vi "svx_Colormap ReplaceState.vi"(9 "Events":T2[](array[typedef])=[enum."[Data] Update"], 10 "RefState":T1={"RefQueue"=refnum, "Properties/Undo"=refnum, "Bound"={"Width"=0, "Height"=0}, "Plot Area:Colors"={"FG Color"=11776947, "BG Color"=0}, "scale legend visible?"=FALSE, "graph palette visible?"=FALSE, "cursor palette visible?"=FALSE, "Ignore Array"=TRUE, "Smooth Update"=FALSE, "Z Scale"={"Z Scale.Scale Fit"=2, "Z Scale.Name Label.Text"="Amplitude", "Z Scale.Interpolate Color"=TRUE, "Visible"=TRUE, "Label Visible"=TRUE, "format string"="%#.2g", "Z Scale.Range"={"Minimum"=0.0, "Maximum"=500.0}}, "X Scale"={"X Scale.Scale Fit"=2, "X Scale.Offset and Multiplier"={"Offset"=0.0, "Multiplier"=1.0}, "X Scale.Name Label.Text"="Time", "X Scale.Range"={"Minimum"=0.0, "Maximum"=10.0}, "Visible"=TRUE, "Label Visible"=TRUE, "format string"="%#.2g"}, "Y Scale"={"Y Scale.Scale Fit"=2, "Y Scale.Offset and Multiplier"={"Offset"=0.0, "Multiplier"=1.0}, "Y Scale.Name Label.Text"="Frequency", "Y Scale.Range"={"Minimum"=0.0, "Maximum"=500.0}, "Visible"=TRUE, "Label Visible"=TRUE, "format string"="%#.2g"}, "Annotation List"=[], "Cursor List"=[], "Display Frequency Lines"=TRUE, "Display Order Lines"=TRUE, "Display Order text"=TRUE, "Display Frequency text"=TRUE, "Order Lineproperty"={"Line"={"Width"=1, "Style"=enum."Dash"}, "color"=0}, "Order Textproperty"={"Test size"=11, "color"=16777222, "background"=16777216}, "Orders"=[], "Frequency"=[], "Frequency Lineproperty"={"Line"={"Width"=1, "Style"=enum."Dash"}, "color"=0}, "Frequency Textproperty"={"Test size"=11, "color"=16777222, "background"=16777216}, "Display Order from Cursor"=FALSE, "Display Freq from Cursor"=FALSE, "Active Cursor"=0, "Selected Cursors"=[], "Cursor Move"=refnum, "Scale Range Change"=refnum}, 11 "NewState":T1={"RefQueue"=refnum, "Properties/Undo"=refnum, "Bound"={"Width"=0, "Height"=0}, "Plot Area:Colors"={"FG Color"=11776947, "BG Color"=0}, "scale legend visible?"=FALSE, "graph palette visible?"=FALSE, "cursor palette visible?"=FALSE, "Ignore Array"=TRUE, "Smooth Update"=FALSE, "Z Scale"={"Z Scale.Scale Fit"=2, "Z Scale.Name Label.Text"="Amplitude", "Z Scale.Interpolate Color"=TRUE, "Visible"=TRUE, "Label Visible"=TRUE, "format string"="%#.2g", "Z Scale.Range"={"Minimum"=0.0, "Maximum"=500.0}}, "X Scale"={"X Scale.Scale Fit"=2, "X Scale.Offset and Multiplier"={"Offset"=0.0, "Multiplier"=1.0}, "X Scale.Name Label.Text"="Time", "X Scale.Range"={"Minimum"=0.0, "Maximum"=10.0}, "Visible"=TRUE, "Label Visible"=TRUE, "format string"="%#.2g"}, "Y Scale"={"Y Scale.Scale Fit"=2, "Y Scale.Offset and Multiplier"={"Offset"=0.0, "Multiplier"=1.0}, "Y Scale.Name Label.Text"="Frequency", "Y Scale.Range"={"Minimum"=0.0, "Maximum"=500.0}, "Visible"=TRUE, "Label Visible"=TRUE, "format string"="%#.2g"}, "Annotation List"=[], "Cursor List"=[], "Display Frequency Lines"=TRUE, "Display Order Lines"=TRUE, "Display Order text"=TRUE, "Display Frequency text"=TRUE, "Order Lineproperty"={"Line"={"Width"=1, "Style"=enum."Dash"}, "color"=0}, "Order Textproperty"={"Test size"=11, "color"=16777222, "background"=16777216}, "Orders"=[], "Frequency"=[], "Frequency Lineproperty"={"Line"={"Width"=1, "Style"=enum."Dash"}, "color"=0}, "Frequency Textproperty"={"Test size"=11, "color"=16777222, "background"=16777216}, "Display Order from Cursor"=FALSE, "Display Freq from Cursor"=FALSE, "Active Cursor"=0, "Selected Cursors"=[], "Cursor Move"=refnum, "Scale Range Change"=refnum}) -> (3 "State out":T1={"RefQueue"=refnum, "Properties/Undo"=refnum, "Bound"={"Width"=0, "Height"=0}, "Plot Area:Colors"={"FG Color"=11776947, "BG Color"=0}, "scale legend visible?"=FALSE, "graph palette visible?"=FALSE, "cursor palette visible?"=FALSE, "Ignore Array"=TRUE, "Smooth Update"=FALSE, "Z Scale"={"Z Scale.Scale Fit"=2, "Z Scale.Name Label.Text"="Amplitude", "Z Scale.Interpolate Color"=TRUE, "Visible"=TRUE, "Label Visible"=TRUE, "format string"="%#.2g", "Z Scale.Range"={"Minimum"=0.0, "Maximum"=500.0}}, "X Scale"={"X Scale.Scale Fit"=2, "X Scale.Offset and Multiplier"={"Offset"=0.0, "Multiplier"=1.0}, "X Scale.Name Label.Text"="Time", "X Scale.Range"={"Minimum"=0.0, "Maximum"=10.0}, "Visible"=TRUE, "Label Visible"=TRUE, "format string"="%#.2g"}, "Y Scale"={"Y Scale.Scale Fit"=2, "Y Scale.Offset and Multiplier"={"Offset"=0.0, "Multiplier"=1.0}, "Y Scale.Name Label.Text"="Frequency", "Y Scale.Range"={"Minimum"=0.0, "Maximum"=500.0}, "Visible"=TRUE, "Label Visible"=TRUE, "format string"="%#.2g"}, "Annotation List"=[], "Cursor List"=[], "Display Frequency Lines"=TRUE, "Display Order Lines"=TRUE, "Display Order text"=TRUE, "Display Frequency text"=TRUE, "Order Lineproperty"={"Line"={"Width"=1, "Style"=enum."Dash"}, "color"=0}, "Order Textproperty"={"Test size"=11, "color"=16777222, "background"=16777216}, "Orders"=[], "Frequency"=[], "Frequency Lineproperty"={"Line"={"Width"=1, "Style"=enum."Dash"}, "color"=0}, "Frequency Textproperty"={"Test size"=11, "color"=16777222, "background"=16777216}, "Display Order from Cursor"=FALSE, "Display Freq from Cursor"=FALSE, "Active Cursor"=0, "Selected Cursors"=[], "Cursor Move"=refnum, "Scale Range Change"=refnum})   [LabVIEW 2017, in "SVX Colormap.xctl"]
uses:
  <vilib>/addons/_XControls/Colormap/SVX Colormap.xctl
  <vilib>/addons/_XControls/Colormap/TypeDef/svx_Colormap_Event.ctl
  <vilib>/addons/_XControls/Colormap/subVIs/svx_Colormap State.ctl
  <vilib>/addons/_XControls/Colormap/TypeDef/svx_Colormap_InnerState.ctl
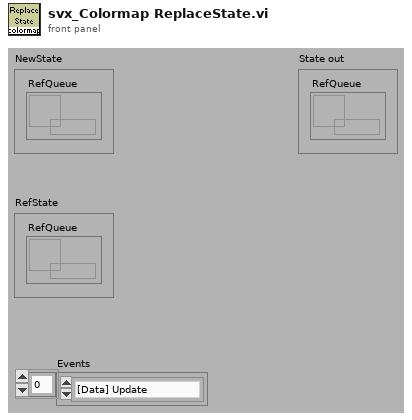
[diagram p1: front panel]
types:
  T1 = typedef "SVX Colormap.xctl/svx_Colormap State.ctl" = cluster{"RefQueue":refnum<queue>, "Properties/Undo":refnum<queue>, "Bound":cluster{"Width":u32, "Height":u32}, "Plot Area:Colors":cluster{"FG Color":u32, "BG Color":u32}, "scale legend visible?":bool, "graph palette visible?":bool, "cursor palette visible?":bool, "Ignore Array":bool, "Smooth Update":bool, "Z Scale":cluster{"Z Scale.Scale Fit":u8, "Z Scale.Name Label.Text":string, "Z Scale.Interpolate Color":bool, "Visible":bool, "Label Visible":bool, "format string":string, "Z Scale.Range":cluster{"Minimum":dbl, "Maximum":dbl}}, "X Scale":cluster{"X Scale.Scale Fit":u8, "X Scale.Offset and Multiplier":cluster{"Offset":dbl, "Multiplier":dbl}, "X Scale.Name Label.Text":string, "X Scale.Range":cluster{"Minimum":dbl, "Maximum":dbl}, "Visible":bool, "Label Visible":bool, "format string":string}, "Y Scale":cluster{"Y Scale.Scale Fit":u8, "Y Scale.Offset and Multiplier":cluster{"Offset":dbl, "Multiplier":dbl}, "Y Scale.Name Label.Text":string, "Y Scale.Range":cluster{"Minimum":dbl, "Maximum":dbl}, "Visible":bool, "Label Visible":bool, "format string":string}, "Annotation List":cluster{"Name":string, "Color":u32, "Style":u8, "Point Style":u8, "Name Visible":bool, "Allow Drag":bool, "Annotation Mode":u32, "Plot":i32, "Index":i32, "Position":cluster{"X":dbl, "Y":dbl}, "X Scale":u32, "Y Scale":u32, "Show Arrow":bool, "Lock Name":bool, "Plot Area":i32, "Label Offset":cluster{"X":dbl, "Y":dbl}}[], "Cursor List":cluster{"Name":string, "Color":u32, "Style":u8, "Point Style":u8, "Name Visible":bool, "Allow Drag":bool, "Cursor Mode":u32, "Plot":i32, "Index":i32, "Position":cluster{"X":dbl, "Y":dbl}, "X Scale":u32, "Y Scale":u32, "Watch Plots":i32[], "Watch All Plots":bool, "Plot Area":i32, "Label Offset":cluster{"X":dbl, "Y":dbl}}[], "Display Frequency Lines":bool, "Display Order Lines":bool, "Display Order text":bool, "Display Frequency text":bool, "Order Lineproperty":cluster{"Line":cluster{"Width":u16, "Style":enum32{"Solid", "Dash", "Dot", "DashDot", "DashDotDot"}}, "color":u32}, "Order Textproperty":cluster{"Test size":i16, "color":u32, "background":u32}, "Orders":dbl[], "Frequency":dbl[], "Frequency Lineproperty":cluster{"Line":cluster{"Width":u16, "Style":enum32{"Solid", "Dash", "Dot", "DashDot", "DashDotDot"}}, "color":u32}, "Frequency Textproperty":cluster{"Test size":i16, "color":u32, "background":u32}, "Display Order from Cursor":bool, "Display Freq from Cursor":bool, "Active Cursor":u32, "Selected Cursors":u32[], "Cursor Move":refnum<user-event>, "Scale Range Change":refnum<user-event>}
  T2 = typedef "SVX Colormap.xctl/svx_Colormap_Event.ctl" = enum16{"None", "[Axis] X Range", "[Axis] Y Range", "[Axis] Z Range", "[Axis] Range", "[Axis] X FString", "[Axis] Y FString", "[Axis] Z FString", "[Axis] X Name", "[Axis] X ScaleVis", "[Axis] X NameVis", "[Axis] Y Name", "[Axis] Y ScaleVis", "[Axis] Y NameVis", "[Axis] Z Name", "[Axis] Z ScaleVis", "[Axis] Z NameVis", "[Image] Line", "[Axis] Z Interp", "[Data] Update", "[Layout] Resize", "[ColorTable] Ignore Array", "[Legend] ScaleVis", "[Legend] GPVis", "[Legend] CPVis", "[Smooth] Update", "[Cursor] Update", "[Plot Area] Colors", "[Size] Minimum", "[Annotation] Update", "[Properties Dialog]", "[Axis] Autoscale X", "[Axis] Autoscale Y", "[Axis] Autoscale Z"}
  T3 = cluster{"Line":cluster{"Width":u16, "Style":enum32{"Solid", "Dash", "Dot", "DashDot", "DashDotDot"}}, "color":u32}
  T4 = cluster{"Test size":i16, "color":u32, "background":u32}
  T5 = cluster{"Name":string, "Color":u32, "Style":u8, "Point Style":u8, "Name Visible":bool, "Allow Drag":bool, "Cursor Mode":u32, "Plot":i32, "Index":i32, "Position":cluster{"X":dbl, "Y":dbl}, "X Scale":u32, "Y Scale":u32, "Watch Plots":i32[], "Watch All Plots":bool, "Plot Area":i32, "Label Offset":cluster{"X":dbl, "Y":dbl}}[]
  T6 = cluster{"Z Scale.Scale Fit":u8, "Z Scale.Name Label.Text":string, "Z Scale.Interpolate Color":bool, "Visible":bool, "Label Visible":bool, "format string":string, "Z Scale.Range":cluster{"Minimum":dbl, "Maximum":dbl}}
  T7 = cluster{"X Scale.Scale Fit":u8, "X Scale.Offset and Multiplier":cluster{"Offset":dbl, "Multiplier":dbl}, "X Scale.Name Label.Text":string, "X Scale.Range":cluster{"Minimum":dbl, "Maximum":dbl}, "Visible":bool, "Label Visible":bool, "format string":string}
  T8 = cluster{"Y Scale.Scale Fit":u8, "Y Scale.Offset and Multiplier":cluster{"Offset":dbl, "Multiplier":dbl}, "Y Scale.Name Label.Text":string, "Y Scale.Range":cluster{"Minimum":dbl, "Maximum":dbl}, "Visible":bool, "Label Visible":bool, "format string":string}
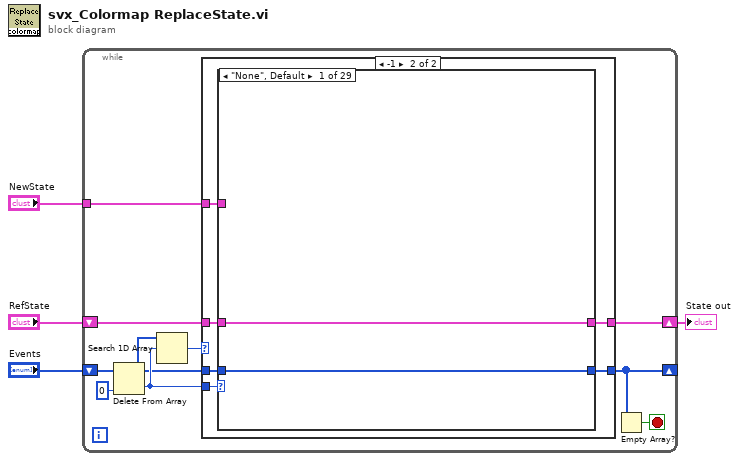
[diagram p0: block diagram]
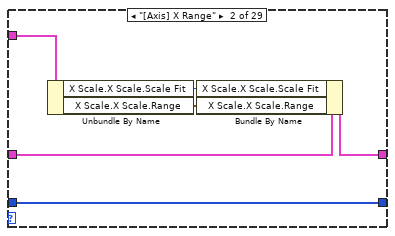
[diagram p3: hidden frame]
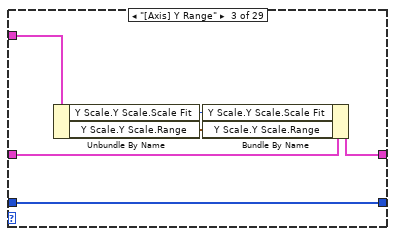
[diagram p4: hidden frame]
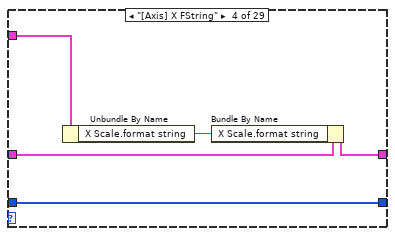
[diagram p5: hidden frame]
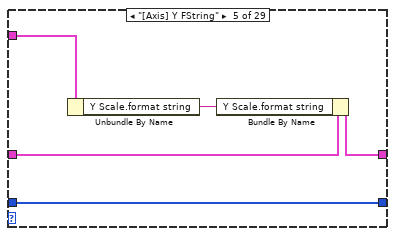
[diagram p6: hidden frame]
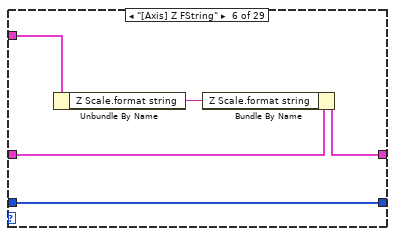
[diagram p7: hidden frame]
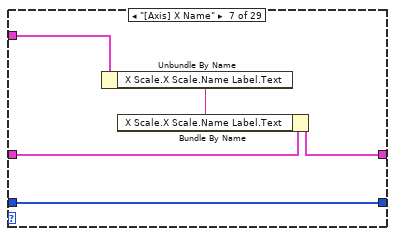
[diagram p8: hidden frame]
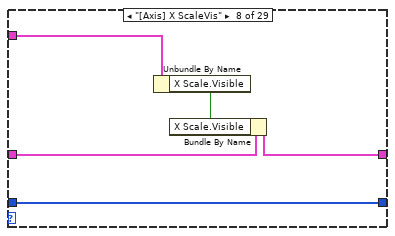
[diagram p9: hidden frame]
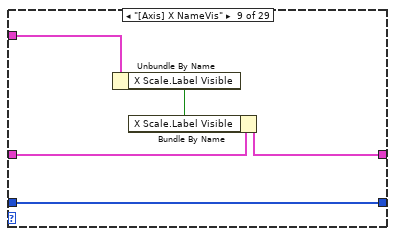
[diagram p10: hidden frame]
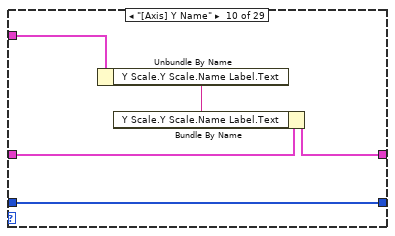
[diagram p11: hidden frame]
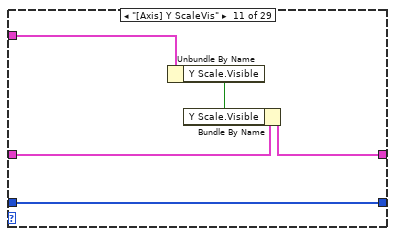
[diagram p12: hidden frame]
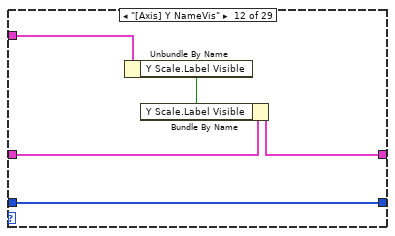
[diagram p13: hidden frame]
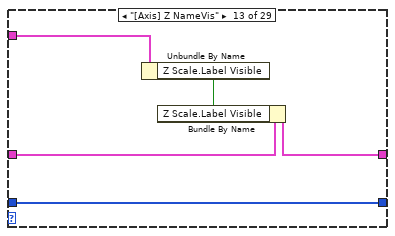
[diagram p14: hidden frame]
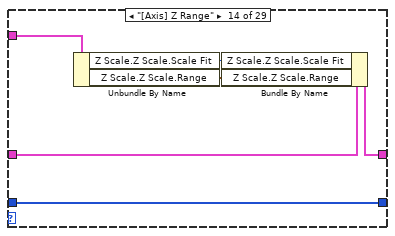
[diagram p15: hidden frame]
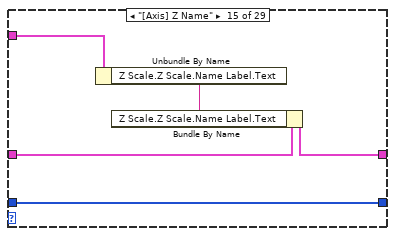
[diagram p16: hidden frame]
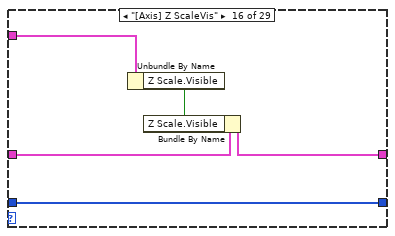
[diagram p17: hidden frame]
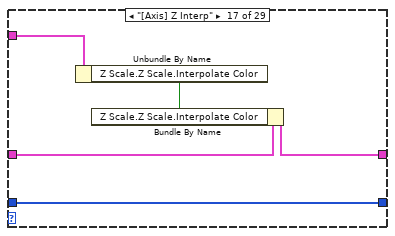
[diagram p18: hidden frame]
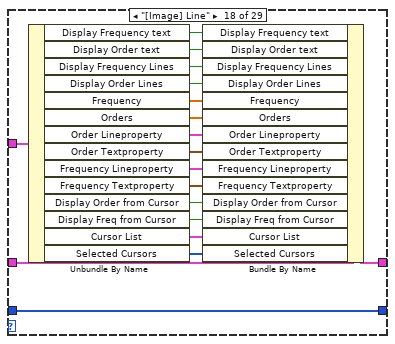
[diagram p19: hidden frame]
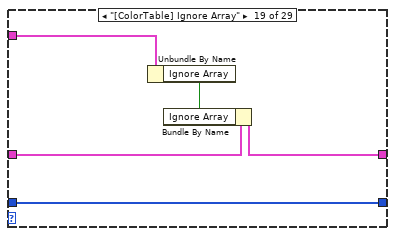
[diagram p20: hidden frame]
diagram:
  n1 = while {
    shift-right: [w9] -> w1
    shift-left: "RefState" -> [w14]
    shift-right: [w11] -> _
    shift-left: "Events" -> [w12]
    tunnel: "NewState" -> [w5]
    stop <- w10 stop-if-true
    n2 = Delete From Array(array=w12, index=0) -> (deleted portion=w8:T2, array with subset deleted=w7:T2[])  [unwired: 1 in]
    n3 = Search 1D Array(1D array=w7, element=w8) -> (index of element=w6:i32)  [unwired: 1 in]
    n4 = case shown="-1" w6 {
      tunnel: w14 -> [w16 w22]
      tunnel: [w15 w21] -> w11
      tunnel: [w16 w20] -> w9
      tunnel: w8 -> [_ w19]
      tunnel: w7 -> [w15 w18]
      tunnel: w5 -> [_ w17]
      frame Default {
      }
      frame -1 {
        n5 = case shown="\"None\", Default" w19 {
          tunnel: w22 -> [w24 w30 w34 w38 w43 w49 w53 w58 w63 w68 w73 w78 w84 w89 w95 w100 w104 w123 w127 w133 w138 w143 w147 w153 w158 w178 w184 w189 w194]
          tunnel: w18 -> [w23 w26 w32 w41 w46 w47 w56 w61 w66 w71 w76 w81 w82 w92 w93 w98 w107 w125 w130 w131 w136 w141 w150 w151 w161 w180 w181 w186 w191]
          tunnel: [w23 w26 w32 w41 w46 w47 w56 w61 w66 w71 w76 w81 w82 w92 w93 w98 w107 w125 w130 w131 w136 w141 w150 w151 w161 w180 w181 w186 w191] -> w21
          tunnel: [w24 w27 w33 w37 w42 w48 w52 w57 w62 w67 w72 w77 w83 w88 w94 w99 w103 w122 w126 w132 w137 w142 w146 w152 w157 w177 w183 w188 w193] -> w20
          tunnel: w17 -> [_ w29 w35 w39 w44 w50 w54 w59 w64 w69 w74 w79 w85 w90 w96 w101 w105 w124 w128 w134 w139 w144 w148 w156 w159 w179 w185 w190 w195]
          frame "None", Default {
          }
          frame "[Axis] X Range" {
            n6 = Unbundle By Name(w29) -> ("X Scale.X Scale.Scale Fit"=w25:u8, "X Scale.X Scale.Range"=w28:cluster{"Minimum":dbl, "Maximum":dbl})
            n7 = Bundle By Name(cluster=w30, "X Scale.X Scale.Scale Fit"=w25, "X Scale.X Scale.Range"=w28) -> (w27:T1)
          }
          frame "[Axis] Y Range" {
            n8 = Unbundle By Name(w35) -> ("Y Scale.Y Scale.Scale Fit"=w31:u8, "Y Scale.Y Scale.Range"=w36:cluster{"Minimum":dbl, "Maximum":dbl})
            n9 = Bundle By Name(cluster=w34, "Y Scale.Y Scale.Scale Fit"=w31, "Y Scale.Y Scale.Range"=w36) -> (w33:T1)
          }
          frame "[Axis] X FString" {
            n10 = Unbundle By Name(w39) -> ("X Scale.format string"=w40:string)
            n11 = Bundle By Name(cluster=w38, "X Scale.format string"=w40) -> (w37:T1)
          }
          frame "[Axis] Y FString" {
            n12 = Unbundle By Name(w44) -> ("Y Scale.format string"=w45:string)
            n13 = Bundle By Name(cluster=w43, "Y Scale.format string"=w45) -> (w42:T1)
          }
          frame "[Axis] Z FString" {
            n14 = Unbundle By Name(w50) -> ("Z Scale.format string"=w51:string)
            n15 = Bundle By Name(cluster=w49, "Z Scale.format string"=w51) -> (w48:T1)
          }
          frame "[Axis] X Name" {
            n16 = Unbundle By Name(w54) -> ("X Scale.X Scale.Name Label.Text"=w55:string)
            n17 = Bundle By Name(cluster=w53, "X Scale.X Scale.Name Label.Text"=w55) -> (w52:T1)
          }
          frame "[Axis] X ScaleVis" {
            n18 = Unbundle By Name(w59) -> ("X Scale.Visible"=w60:bool)
            n19 = Bundle By Name(cluster=w58, "X Scale.Visible"=w60) -> (w57:T1)
          }
          frame "[Axis] X NameVis" {
            n20 = Unbundle By Name(w64) -> ("X Scale.Label Visible"=w65:bool)
            n21 = Bundle By Name(cluster=w63, "X Scale.Label Visible"=w65) -> (w62:T1)
          }
          frame "[Axis] Y Name" {
            n22 = Unbundle By Name(w69) -> ("Y Scale.Y Scale.Name Label.Text"=w70:string)
            n23 = Bundle By Name(cluster=w68, "Y Scale.Y Scale.Name Label.Text"=w70) -> (w67:T1)
          }
          frame "[Axis] Y ScaleVis" {
            n24 = Unbundle By Name(w74) -> ("Y Scale.Visible"=w75:bool)
            n25 = Bundle By Name(cluster=w73, "Y Scale.Visible"=w75) -> (w72:T1)
          }
          frame "[Axis] Y NameVis" {
            n26 = Unbundle By Name(w79) -> ("Y Scale.Label Visible"=w80:bool)
            n27 = Bundle By Name(cluster=w78, "Y Scale.Label Visible"=w80) -> (w77:T1)
          }
          frame "[Axis] Z NameVis" {
            n28 = Unbundle By Name(w85) -> ("Z Scale.Label Visible"=w86:bool)
            n29 = Bundle By Name(cluster=w84, "Z Scale.Label Visible"=w86) -> (w83:T1)
          }
          frame "[Axis] Z Range" {
            n30 = Unbundle By Name(w90) -> ("Z Scale.Z Scale.Scale Fit"=w87:u8, "Z Scale.Z Scale.Range"=w91:cluster{"Minimum":dbl, "Maximum":dbl})
            n31 = Bundle By Name(cluster=w89, "Z Scale.Z Scale.Scale Fit"=w87, "Z Scale.Z Scale.Range"=w91) -> (w88:T1)
          }
          frame "[Axis] Z Name" {
            n32 = Unbundle By Name(w96) -> ("Z Scale.Z Scale.Name Label.Text"=w97:string)
            n33 = Bundle By Name(cluster=w95, "Z Scale.Z Scale.Name Label.Text"=w97) -> (w94:T1)
          }
          frame "[Axis] Z ScaleVis" {
            n34 = Unbundle By Name(w101) -> ("Z Scale.Visible"=w102:bool)
            n35 = Bundle By Name(cluster=w100, "Z Scale.Visible"=w102) -> (w99:T1)
          }
          frame "[Axis] Z Interp" {
            n36 = Unbundle By Name(w105) -> ("Z Scale.Z Scale.Interpolate Color"=w106:bool)
            n37 = Bundle By Name(cluster=w104, "Z Scale.Z Scale.Interpolate Color"=w106) -> (w103:T1)
          }
          frame "[Image] Line" {
            n38 = Unbundle By Name(w124) -> ("Display Frequency text"=w121:bool, "Display Order text"=w120:bool, "Display Frequency Lines"=w119:bool, "Display Order Lines"=w118:bool, "Frequency"=w117:dbl[], "Orders"=w116:dbl[], "Order Lineproperty"=w115:T3, "Order Textproperty"=w114:T4, "Frequency Lineproperty"=w113:T3, "Frequency Textproperty"=w112:T4, "Display Order from Cursor"=w108:bool, "Display Freq from Cursor"=w109:bool, "Cursor List"=w111:T5, "Selected Cursors"=w110:u32[])
            n39 = Bundle By Name(cluster=w123, "Display Frequency text"=w121, "Display Order text"=w120, "Display Frequency Lines"=w119, "Display Order Lines"=w118, "Frequency"=w117, "Orders"=w116, "Order Lineproperty"=w115, "Order Textproperty"=w114, "Frequency Lineproperty"=w113, "Frequency Textproperty"=w112, "Display Order from Cursor"=w108, "Display Freq from Cursor"=w109, "Cursor List"=w111, "Selected Cursors"=w110) -> (w122:T1)
          }
          frame "[ColorTable] Ignore Array" {
            n40 = Unbundle By Name(w128) -> ("Ignore Array"=w129:bool)
            n41 = Bundle By Name(cluster=w127, "Ignore Array"=w129) -> (w126:T1)
          }
          frame "[Legend] ScaleVis" {
            n42 = Unbundle By Name(w134) -> ("scale legend visible?"=w135:bool)
            n43 = Bundle By Name(cluster=w133, "scale legend visible?"=w135) -> (w132:T1)
          }
          frame "[Legend] GPVis" {
            n44 = Unbundle By Name(w139) -> ("graph palette visible?"=w140:bool)
            n45 = Bundle By Name(cluster=w138, "graph palette visible?"=w140) -> (w137:T1)
          }
          frame "[Legend] CPVis" {
            n46 = Unbundle By Name(w144) -> ("cursor palette visible?"=w145:bool)
            n47 = Bundle By Name(cluster=w143, "cursor palette visible?"=w145) -> (w142:T1)
          }
          frame "[Smooth] Update" {
            n48 = Unbundle By Name(w148) -> ("Smooth Update"=w149:bool)
            n49 = Bundle By Name(cluster=w147, "Smooth Update"=w149) -> (w146:T1)
          }
          frame "[Cursor] Update" {
            n50 = Unbundle By Name(w156) -> ("Cursor List"=w155:T5, "Selected Cursors"=w154:u32[])
            n51 = Bundle By Name(cluster=w153, "Cursor List"=w155, "Selected Cursors"=w154) -> (w152:T1)
          }
          frame "[Plot Area] Colors" {
            n52 = Unbundle By Name(w159) -> ("Plot Area:Colors"=w160:cluster{"FG Color":u32, "BG Color":u32})
            n53 = Bundle By Name(cluster=w158, "Plot Area:Colors"=w160) -> (w157:T1)
          }
          frame "[Properties Dialog]" {
            n54 = Unbundle By Name(w179) -> ("Z Scale"=w176:T6, "X Scale"=w175:T7, "Y Scale"=w174:T8, "Display Frequency Lines"=w173:bool, "Display Order Lines"=w172:bool, "Display Order text"=w171:bool, "Display Frequency text"=w170:bool, "Order Lineproperty"=w169:T3, "Order Textproperty"=w168:T4, "Orders"=w167:dbl[], "Frequency"=w166:dbl[], "Frequency Lineproperty"=w165:T3, "Frequency Textproperty"=w164:T4, "Display Order from Cursor"=w163:bool, "Display Freq from Cursor"=w162:bool)
            n55 = Bundle By Name(cluster=w178, "Z Scale"=w176, "X Scale"=w175, "Y Scale"=w174, "Display Frequency Lines"=w173, "Display Order Lines"=w172, "Display Order text"=w171, "Display Frequency text"=w170, "Order Lineproperty"=w169, "Order Textproperty"=w168, "Orders"=w167, "Frequency"=w166, "Frequency Lineproperty"=w165, "Frequency Textproperty"=w164, "Display Order from Cursor"=w163, "Display Freq from Cursor"=w162) -> (w177:T1)
          }
          frame "[Axis] Autoscale X" {
            n56 = Unbundle By Name(w185) -> ("X Scale.X Scale.Scale Fit"=w182:u8)
            n57 = Bundle By Name(cluster=w184, "X Scale.X Scale.Scale Fit"=w182) -> (w183:T1)
          }
          frame "[Axis] Autoscale Y" {
            n58 = Unbundle By Name(w190) -> ("Y Scale.Y Scale.Scale Fit"=w187:u8)
            n59 = Bundle By Name(cluster=w189, "Y Scale.Y Scale.Scale Fit"=w187) -> (w188:T1)
          }
          frame "[Axis] Autoscale Z" {
            n60 = Unbundle By Name(w195) -> ("Z Scale.Z Scale.Scale Fit"=w192:u8)
            n61 = Bundle By Name(cluster=w194, "Z Scale.Z Scale.Scale Fit"=w192) -> (w193:T1)
          }
        }
      }
    }
    n62 = Empty Array?(array=w11) -> (empty?=w10:bool)
  }
  "State out" <- w1
